vi "Normalized Case.vi"(0 "m":u32[](array[numeric]), 1 "n-m":u32[](array[numeric]), 2 "table":dbl[][](array[numeric]) format="%.2f") -> (3 "m*":u32[](array[numeric]), 4 "n-m*":u32[](array[numeric]), 5 "table*":dbl[][](array[numeric]) format="%.2f", 6 "error":i32)   [LabVIEW 2010, in "NI_Gmath.lvlib"]
uses:
  NI_Gmath.lvlib
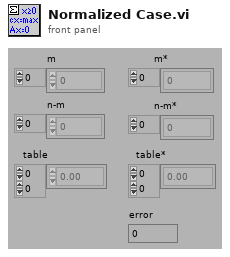
[diagram p1: front panel]
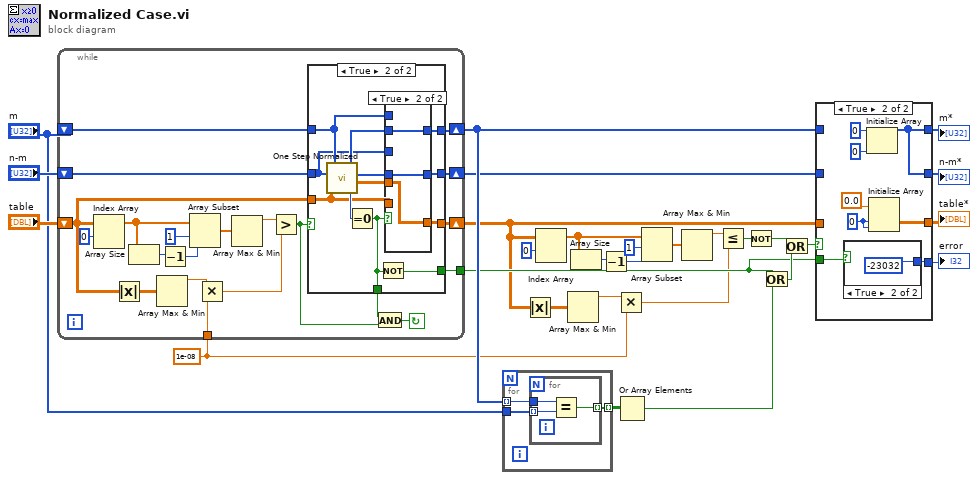
[diagram p0: block diagram]
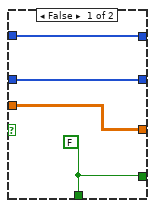
[diagram p2: hidden frame]
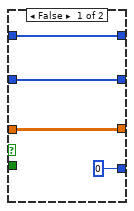
[diagram p4: hidden frame]
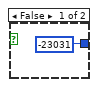
[diagram p5: hidden frame]
diagram:
  w2 = 1e-08
  n1 = while {
    tunnel: w2 -> [w30]
    tunnel: [w39] -> w7
    shift-left: "table" -> [w33]
    shift-right: [w38] -> w4
    shift-left: "n-m" -> [w42]
    shift-right: [w36] -> w22
    shift-left: "m" -> [w43]
    shift-right: [w37] -> w24
    stop <- w40 continue-if-true
    n2 = Index Array(array=w33, index (row)=0) -> (element=w47:dbl[])  [unwired: 1 in]
    n3 = Absolute Value(x=w33) -> (abs(x)=w32:dbl[][])
    n4 = Array Size(array=w47) -> (size(s)=w46:i32)
    n5 = Array Max & Min(array=w32) -> (max value=w31:dbl)  [unwired: 3 out]
    n6 = Decrement(x=w46) -> (x-1=w45:i32)
    n7 = Array Subset(array=w47, index=1, length=w45) -> (w44:dbl[])
    n8 = Multiply(x=w31, y=w30) -> (x*y=w29:dbl)
    n9 = Array Max & Min(array=w44) -> (max value=w34:dbl)  [unwired: 3 out]
    n10 = Greater?(x=w34, y=w29) -> (0:w35:bool)
    n11 = case shown="True" w35 {
      tunnel: w43 -> [w53 w58]
      tunnel: [w53 w63] -> w37
      tunnel: w33 -> [w52 w56]
      tunnel: [w52 w59] -> w38
      tunnel: w42 -> [w51 w57]
      tunnel: [w51 w61] -> w36
      tunnel: [w50 w55] -> w41
      tunnel: [w50 w54] -> w39
      frame False {
        w50 = FALSE
      }
      frame True {
        n12 = call "One Step Normalized.vi"("m"=w58, "n-m"=w57, "table"=w56) -> ("m*"=w64:u32[], "n-m*"=w62:u32[], "table*"=w60:dbl[][], "error"=w65:i32)
        n13 = Equal To 0?(x=w65) -> (x = 0?=w55:bool)
        n14 = Not(x=w55) -> (.not. x?=w54:bool)
        n15 = case shown="True" w55 {
          tunnel: w64 -> [_ w71]
          tunnel: [w68 w71] -> w63
          tunnel: w62 -> [_ w70]
          tunnel: [w67 w70] -> w61
          tunnel: w60 -> [_ w69]
          tunnel: [w66 w69] -> w59
          tunnel: w58 -> [w68 _]
          tunnel: w57 -> [w67 _]
          tunnel: w56 -> [w66 _]
          frame False {
          }
          frame True {
          }
        }
      }
    }
    n16 = And(x=w41, y=w35) -> (x .and. y?=w40:bool)
  }
  n17 = for {
    tunnel: w24 -> [w74] mode=indexing
    tunnel: "m" -> [w73]
    tunnel: [w72] -> w25 mode=indexing
    n18 = for {
      tunnel: w74 -> [w77]
      tunnel: w73 -> [w76] mode=indexing
      tunnel: [w75] -> w72 mode=indexing
      n19 = Equal?(x=w77, y=w76) -> (x = y?=w75:bool)
    }
  }
  n20 = Absolute Value(x=w4) -> (abs(x)=w5:dbl[][])
  n21 = Index Array(array=w4, index (row)=0) -> (element=w16:dbl[])  [unwired: 1 in]
  n22 = Array Max & Min(array=w5) -> (max value=w3:dbl)  [unwired: 3 out]
  n23 = Array Size(array=w16) -> (size(s)=w15:i32)
  n24 = Decrement(x=w15) -> (x-1=w14:i32)
  n25 = Multiply(x=w3, y=w2) -> (x*y=w1:dbl)
  n26 = Or Array Elements(Boolean array=w25) -> (logical OR=w6:bool)
  n27 = Array Subset(array=w16, index=1, length=w14) -> (w13:dbl[])
  n28 = Array Max & Min(array=w13) -> (max value=w9:dbl)  [unwired: 3 out]
  n29 = Less Or Equal?(x=w9, y=w1) -> (x <= y?=w12:bool)
  n30 = Not(x=w12) -> (.not. x?=w8:bool)
  n31 = Or(x=w7, y=w6) -> (x .or. y?=w11:bool)
  n32 = Or(x=w8, y=w11) -> (x .or. y?=w10:bool)
  n33 = case shown="True" w10 {
    tunnel: w24 -> [w81 _]
    tunnel: [w81 w87] -> w23
    tunnel: w22 -> [w80 _]
    tunnel: [w80 w87] -> w21
    tunnel: [0 w89] -> w20
    tunnel: [w78 w83] -> w19
    tunnel: w4 -> [w78 _]
    tunnel: w7 -> [_ w82]
    frame False {
    }
    frame True {
      w85 = 0
      n34 = case shown="True" w82 {
        tunnel: [-23031 -23032] -> w89
        frame False {
        }
        frame True {
        }
      }
      n35 = Initialize Array(u32 0, 0) -> (w87:u32[])
      n36 = Initialize Array(0.0, w85, w85) -> (w83:dbl[][])
    }
  }
  "n-m*" <- w21
  "m*" <- w23
  "error" <- w20
  "table*" <- w19
